vi "restore_project_item.vi"(8 "error in (no error)":errorcluster, 11 "ProjectItem in":refnum<vi>) -> (0 "error out":errorcluster, 3 "ProjectItem out":refnum<vi>)   [LabVIEW 2019, in "Conditional Disable Build Actions.lvlib"]
uses:
  Conditional Disable Build Actions.lvlib
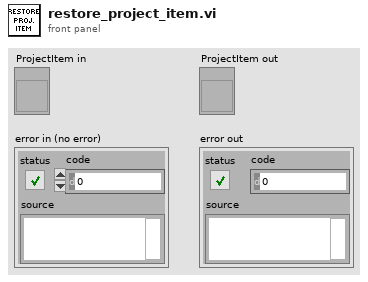
[diagram p1: front panel]
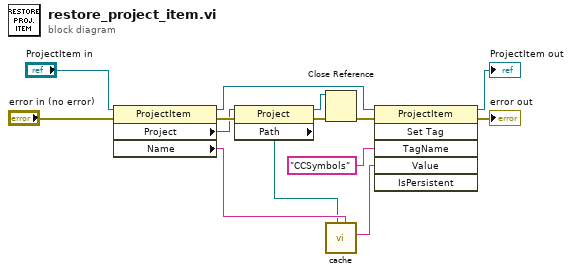
[diagram p0: block diagram]
diagram:
  n1 = property class="ProjectItem"(reference="ProjectItem in", error in="error in (no error)") -> (reference out=w6:refnum<vi>, error out=w9:errorcluster, "Project"=w8:refnum<vi>, "Name"=w11:string)
  n2 = property class="Project"(reference=w8, error in=w9) -> (reference out=w12:refnum<vi>, error out=w13:errorcluster, "Path"=w10:path)
  n3 = Close Reference(reference=w12, error in (no error)=w13) -> (error out=w14:errorcluster)
  n4 = call "cache.vi"("target"=w11, "project path"=w10) -> ("CCSymbols out"=w4:string)  [unwired: 9 in]
  n5 = invoke class="ProjectItem" method="Set Tag"(reference=w6, error in=w14, "TagName"="CCSymbols" ("Tag Name"), "Value"=w4) -> (reference out=→"ProjectItem out":refnum<vi>, error out=→"error out":errorcluster)  [unwired: 2 in, 4 out]
